vi "Shift_image.vi"(6 "Mask Level: Ref smaller is Black":i32=150, 8 "Relative y-Jitter":i32=9, 9 "Exchange X and Y":bool, 10 "Reference image c0":i32[][](graph), 11 "Data image":i32[][](graph)) -> (3 "Data / Ref with Jitter_correction":dbl[][](graph))   [LabVIEW 2014]
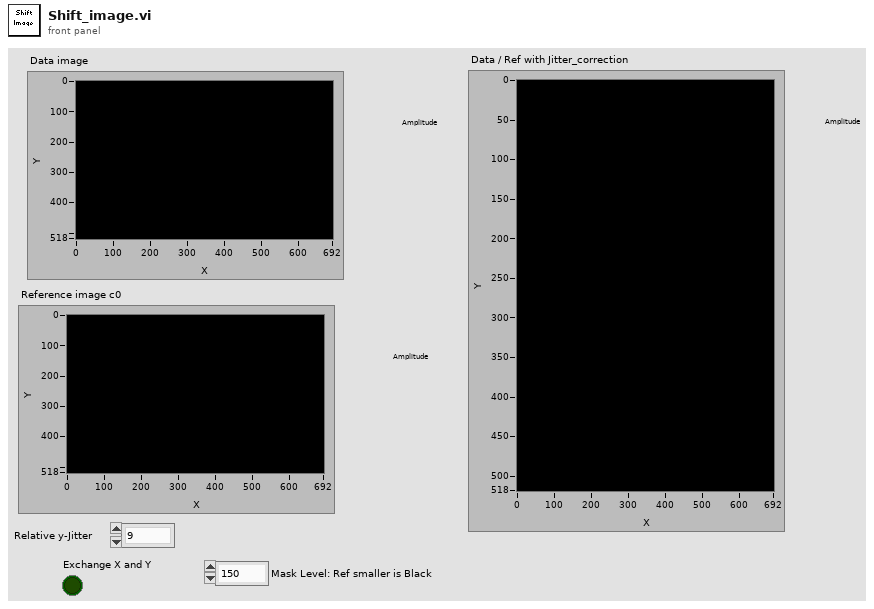
[diagram p1: front panel]
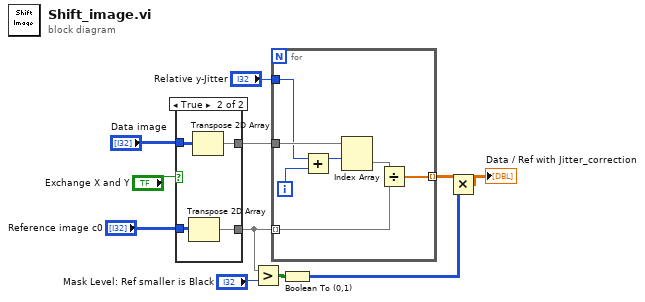
[diagram p0: block diagram]
diagram:
  n1 = case shown="True" "Exchange X and Y" {
    tunnel: "Data image" -> [w13 w17]
    tunnel: [w13 w16] -> w10
    tunnel: "Reference image c0" -> [w12 w15]
    tunnel: [w12 w14] -> w5
    frame False {
    }
    frame True {
      n2 = Transpose 2D Array(2D array=w15) -> (transposed array=w14:i32[][])
      n3 = Transpose 2D Array(2D array=w17) -> (transposed array=w16:i32[][])
    }
  }
  n4 = Greater?(x=w5, y="Mask Level: Ref smaller is Black") -> (0:w4:bool[][])
  n5 = for {
    tunnel: w10 -> [w24]
    tunnel: w5 -> [w20] mode=indexing
    tunnel: "Relative y-Jitter" -> [w21]
    tunnel: [w18] -> w3 mode=indexing
    i -> [w22]
    n6 = Add(x=w21, y=w22) -> (x+y=w23:i32)
    n7 = Index Array(array=w24, index (row)=w23) -> (element=w19:i32[])  [unwired: 1 in]
    n8 = Divide(x=w19, y=w20) -> (x/y=w18:dbl[])
  }
  n9 = Boolean To (0,1)(Boolean=w4) -> (0, 1=w2:i16[][])
  n10 = Multiply(x=w3, y=w2) -> (x*y=→"Data / Ref with Jitter_correction":dbl[][])
